vi "ERIO WIN Process State Variables.vi"(6 "Supervisory Variables In":T3={"Alarm Threshold"=0.0, "Shutdown"=FALSE, "Enable SNS Alarm"=FALSE, "Enable SNS Stage Notification"=FALSE, "Enable SQS Notification"=FALSE, "Enable S3 TDMS Signal Capture"=FALSE, "Enable SystemLink Signal Capture"=FALSE, "Capture Signal"=FALSE, "Server Update"=FALSE, "AWS Access Key"="AKIAINLDO2Y2PDFEWDOQ", "AWS Secret Key"="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", "Phone Number"="+15037066913", "Region"=enum."us-west-2", "AWS SQS Queue"="+15037066913", "AWS S3 Bucket"="+15037066913"}, 7 "WIN State In":T1, 8 "error in (no error)":errorcluster, 9 "AWS Variables In":T5, 11 "EEISysLink.lvclass In":refnum<class "EEISysLink.lvclass">) -> (0 "error out":errorcluster, 1 "AWS Variables Out":T5, 3 "EEISysLink.lvclass Out":refnum<class "EEISysLink.lvclass">, 4 "Supervisory Variables Out":T3={"Alarm Threshold"=0.0, "Shutdown"=FALSE, "Enable SNS Alarm"=FALSE, "Enable SNS Stage Notification"=FALSE, "Enable SQS Notification"=FALSE, "Enable S3 TDMS Signal Capture"=FALSE, "Enable SystemLink Signal Capture"=FALSE, "Capture Signal"=FALSE, "Server Update"=FALSE, "AWS Access Key"="AKIAINLDO2Y2PDFEWDOQ", "AWS Secret Key"="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", "Phone Number"="+15037066913", "Region"=enum."us-west-2", "AWS SQS Queue"="+15037066913", "AWS S3 Bucket"="+15037066913"}, 5 "WIN State Out":T1)   [LabVIEW 2017]
doc: "Process conveyor simulation state variables on Windows supervisor program. Update process variables on the SystemLink server and then pass downstream for supervisory processing. \n\nJames Tillett P.E.\nEndeavor Engineering Inc.\nwww.endeavoreng.com"
uses:
  Class EEISysLink/EEISysLink.lvclass
  Controls/ERIO AWS Toolkit Variables.ctl
  <vilib>/AWS Toolkit/SQS/Queue/Queue.lvclass
  <vilib>/AWS Toolkit/SNS/Phone Number/Phone Number.lvclass
  <vilib>/AWS Toolkit/S3/Bucket/Bucket.lvclass
  Controls/ERIO Supervisory Variables.ctl
  <vilib>/AWS Toolkit/Core/HTTP Request/Region.ctl
  Controls/ERIO WIN State Variables.ctl
  Controls/ERIO Worker Variables.ctl
  Class EEISysLink/Controls/SL Tag Scope.ctl
  Class EEISysLink/Controls/SL Tag Type.ctl
  <vilib>/AWS Toolkit/Core/HTTP Request/HTTP Request.lvclass
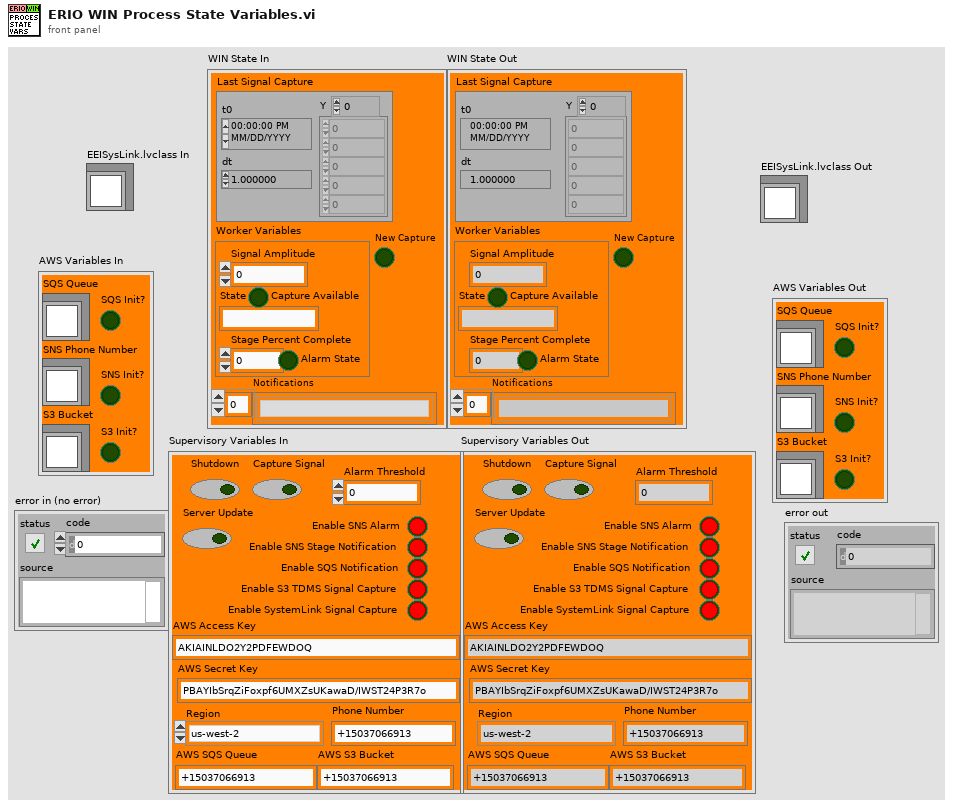
[diagram p1: front panel]
types:
  T1 = typedef "ERIO WIN State Variables.ctl" = cluster{"Worker Variables":T2, "Notifications":string[], "New Capture":bool, "Last Signal Capture":waveform(dbl)}
  T2 = typedef "ERIO Worker Variables.ctl" = cluster{"Signal Amplitude":dbl, "State":string, "Stage Percent Complete":dbl, "Alarm State":bool, "Capture Available":bool}
  T3 = typedef "ERIO Supervisory Variables.ctl" = cluster{"Alarm Threshold":dbl, "Shutdown":bool, "Enable SNS Alarm":bool, "Enable SNS Stage Notification":bool, "Enable SQS Notification":bool, "Enable S3 TDMS Signal Capture":bool, "Enable SystemLink Signal Capture":bool, "Capture Signal":bool, "Server Update":bool, "AWS Access Key":string, "AWS Secret Key":string, "Phone Number":string, "Region":T4, "AWS SQS Queue":string, "AWS S3 Bucket":string}
  T4 = typedef "NI_AWS_Core.lvlib/HTTP Request.lvclass/Region.ctl" = enum16{"us-east-1", "us-east-2", "us-west-1", "us-west-2", "ap-northeast-1", "ap-northeast-2", "ap-southeast-1", "ap-southeast-2", "ca-central-1", "eu-central-1", "eu-west-1", "eu-west-2", "sa-east-1"}
  T5 = typedef "ERIO AWS Toolkit Variables.ctl" = cluster{"SQS Queue":refnum<class "Queue.lvclass">, "SNS Phone Number":refnum<class "Phone Number.lvclass">, "S3 Bucket":refnum<class "Bucket.lvclass">, "SQS Init?":bool, "S3 Init?":bool, "SNS Init?":bool}
  T6 = typedef "EEISysLink.lvclass/SL Tag Type.ctl" = enum16{"All", "Supervisor", "Worker"}
  T7 = typedef "EEISysLink.lvclass/SL Tag Scope.ctl" = enum16{"Local", "Server"}
  T8 = typedef "SL Tag Value.ctl" = cluster{"Value":variant, "Time Stamp":timestamp, "Tag Data Type":T9, "Name":string}
  T9 = typedef "EEISysLink.lvclass/SL Tag Data Type.ctl" = enum16{"Double", "Integer", "String", "Boolean", "Waveform"}
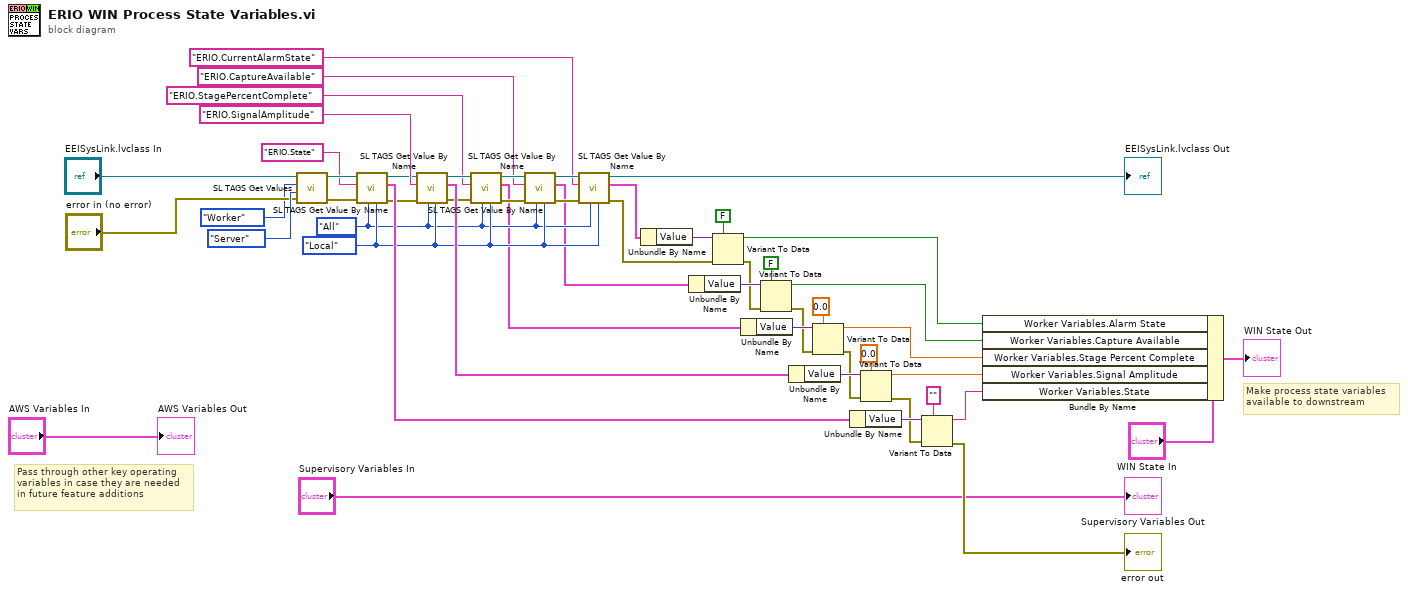
[diagram p0: block diagram]
diagram:
  w15 = SL_Tag_Type."All" ("Tag Type")
  w16 = SL_Tag_Scope."Local" ("Tag Scope")
  # "Make process state variables \navailable to downstream"
  # "Pass through other key operating\nvariables in case they are needed\nin future feature additions"
  n1 = call-dynamic "SL TAGS Get Values.vi"("error in (no error)"="error in (no error)", "Tag Scope"=SL_Tag_Scope."Server", "Tag Type"=SL_Tag_Type."Worker", "EEISysLink in"="EEISysLink.lvclass In") -> ("error out"=w51:errorcluster, "EEISysLink out"=w50:refnum<class "EEISysLink.lvclass">)  [unwired: 5 in, 1 out]
  n2 = call-dynamic "SL TAGS Get Value By Name.vi"("Tag Scope"=w16, "Tag Type"=w15, "error in (no error)"=w51, "Tag Name"="ERIO.State", "EEISysLink in"=w50) -> ("error out"=w1:errorcluster, "Tag Value"=w40:T8, "EEISysLink out"=w2:refnum<class "EEISysLink.lvclass">)  [unwired: 3 in, 1 out]
  n3 = call-dynamic "SL TAGS Get Value By Name.vi"("Tag Scope"=w16, "Tag Type"=w15, "error in (no error)"=w1, "Tag Name"="ERIO.SignalAmplitude", "EEISysLink in"=w2) -> ("error out"=w28:errorcluster, "Tag Value"=w41:T8, "EEISysLink out"=w32:refnum<class "EEISysLink.lvclass">)  [unwired: 3 in, 1 out]
  n4 = call-dynamic "SL TAGS Get Value By Name.vi"("Tag Scope"=w16, "Tag Type"=w15, "error in (no error)"=w28, "Tag Name"="ERIO.StagePercentComplete", "EEISysLink in"=w32) -> ("error out"=w18:errorcluster, "Tag Value"=w12:T8, "EEISysLink out"=w20:refnum<class "EEISysLink.lvclass">)  [unwired: 3 in, 1 out]
  n5 = call-dynamic "SL TAGS Get Value By Name.vi"("Tag Scope"=w16, "Tag Type"=w15, "error in (no error)"=w18, "Tag Name"="ERIO.CaptureAvailable", "EEISysLink in"=w20) -> ("error out"=w17:errorcluster, "Tag Value"=w11:T8, "EEISysLink out"=w21:refnum<class "EEISysLink.lvclass">)  [unwired: 3 in, 1 out]
  n6 = call-dynamic "SL TAGS Get Value By Name.vi"("Tag Scope"=w16, "Tag Type"=w15, "error in (no error)"=w17, "Tag Name"="ERIO.CurrentAlarmState", "EEISysLink in"=w21) -> ("error out"=w9:errorcluster, "Tag Value"=w10:T8, "EEISysLink out"=→"EEISysLink.lvclass Out":refnum<class "EEISysLink.lvclass">)  [unwired: 3 in, 1 out]
  n7 = Unbundle By Name(w10) -> ("Value"=w24:variant)
  n8 = Unbundle By Name(w11) -> ("Value"=w23:variant)
  n9 = Variant To Data(error in=w9, type=FALSE, Variant=w24) -> (data=w5:bool, error out=w8:errorcluster)
  n10 = Unbundle By Name(w12) -> ("Value"=w30:variant)
  n11 = Variant To Data(error in=w8, type=FALSE, Variant=w23) -> (data=w6:bool, error out=w7:errorcluster)
  n12 = Unbundle By Name(w41) -> ("Value"=w43:variant)
  n13 = Variant To Data(error in=w7, type=0.0, Variant=w30) -> (data=w27:dbl, error out=w26:errorcluster)
  n14 = Unbundle By Name(w40) -> ("Value"=w42:variant)
  n15 = Variant To Data(error in=w26, type=0.0, Variant=w43) -> (data=w38:dbl, error out=w3:errorcluster)
  n16 = Variant To Data(error in=w3, type="", Variant=w42) -> (data=w37:string, error out=→"error out":errorcluster)
  n17 = Bundle By Name(cluster="WIN State In", "Worker Variables.Alarm State"=w5, "Worker Variables.Capture Available"=w6, "Worker Variables.Stage Percent Complete"=w27, "Worker Variables.Signal Amplitude"=w38, "Worker Variables.State"=w37) -> (→"WIN State Out":T1)
  "AWS Variables Out" <- "AWS Variables In"
  "Supervisory Variables Out" <- "Supervisory Variables In"
